vi "Elevate.vi"(9 "Power":dbl, 10 "Reverse?":bool) -> ()   [LabVIEW 2017]
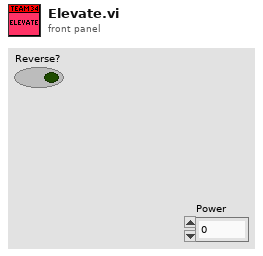
[diagram p1: front panel]
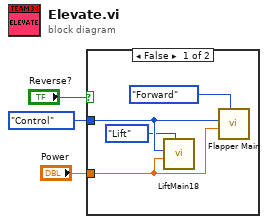
[diagram p0: block diagram]
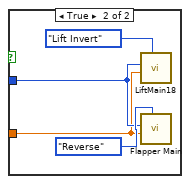
[diagram p2: hidden frame]
diagram:
  n1 = case shown="False" "Reverse?" {
    tunnel: enum16{"Open", "Control"}."Control" ("Control Mode") -> [w7 w9]
    tunnel: "Power" -> [w4 w8]
    frame False {
      n2 = call "LiftMain18.vi"("Operation Mode"=enum16{"Lift", "Lift Invert", "Zero"}."Lift", "Power"=w4, "Control Mode"=w7) -> ()  [unwired: 9 in]
      n3 = call "Flapper Main.vi"("Control Options"=enum16{"Zero", "Forward", "Reverse"}."Forward", "Power"=w4, "Control Mode"=w7) -> ()  [unwired: 9 in]
    }
    frame True {
      n4 = call "LiftMain18.vi"("Operation Mode"=enum16{"Lift", "Lift Invert", "Zero"}."Lift Invert", "Power"=w8, "Control Mode"=w9) -> ()  [unwired: 9 in]
      n5 = call "Flapper Main.vi"("Control Options"=enum16{"Zero", "Forward", "Reverse"}."Reverse", "Power"=w8, "Control Mode"=w9) -> ()  [unwired: 9 in]
    }
  }
